vi "Lvi Read U32Data2D.vi"(0 "DataBufSize":u32, 1 "timeout":dbl, 5 "TaskRef":i32, 7 "PointsPerChan":u32, 9 "NumChansToRead":u32, 11 "error in (no error)":errorcluster, 12 "OnlyReadAvailable":bool) -> (3 "DataBuf":u32[](array[numeric]), 4 "DataBufSize out":u32, 6 "TaskRef out":i32, 8 "PointsPerChan out":u32, 10 "NumChansToRead out":u32, 14 "function return":i32, 15 "error out":errorcluster)   [LabVIEW 2022 SP3, in "DtLvLink.lvlib"]
doc: "Calls directly into the entry points of the DLL of the Data Acq SDK to return a two-dimensional array of unsigned, 32-bit integers representing the data points from the specified task."
uses:
  DtLvLink.lvlib
  <userlib>/LV-Link3/DtLvLink_64.dll
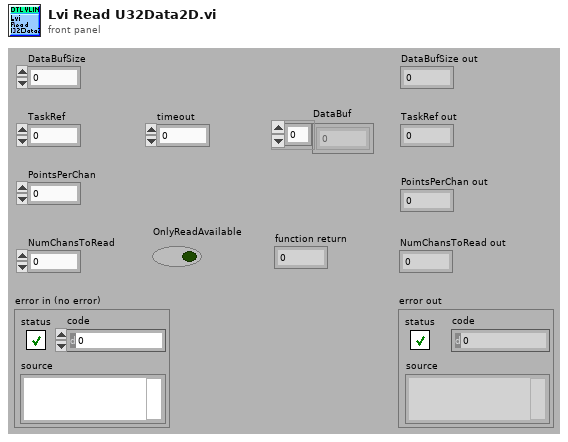
[diagram p1: front panel]
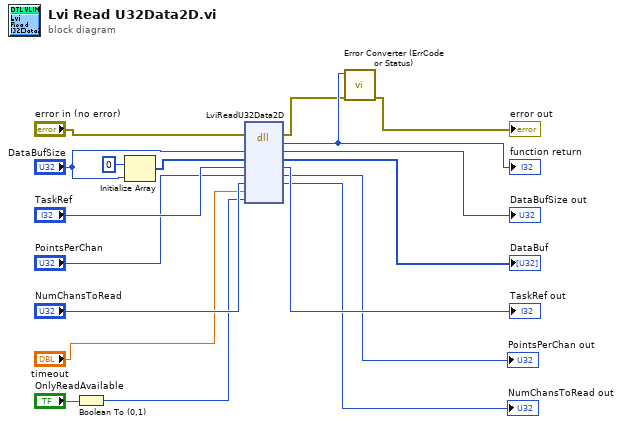
[diagram p0: block diagram]
diagram:
  n1 = Boolean To (0,1)(Boolean="OnlyReadAvailable") -> (0, 1=w3:i16)
  n2 = Initialize Array(u32 0 ("element"), "DataBufSize") -> (w15:u32[])
  n3 = dll-call lib="C:/Program Files/National Instruments/LabVIEW 2022/user.lib/LV-Link3/DtLvLink_64.*" fn="LviReadU32Data2D"(error in="error in (no error)", "DataBufSize"="DataBufSize", "DataBuf"=w15, "TaskRef"="TaskRef", "PointsPerChan"="PointsPerChan", "NumChansToRead"="NumChansToRead", "timeout"="timeout", "OnlyReadAvailable"=w3) -> (error out=w6:errorcluster, "return type"=w18:i32, "DataBufSize"=→"DataBufSize out":u32, "DataBuf"=→"DataBuf":u32[], "TaskRef"=→"TaskRef out":i32, "PointsPerChan"=→"PointsPerChan out":u32, "NumChansToRead"=→"NumChansToRead out":u32)  [unwired: 4 in, 1 out]
  "function return" <- w18
  n4 = call "Error Converter (ErrCode or Status).vi"("error in (no error)"=w6, "error code"=w18) -> ("error out"=→"error out":errorcluster)  [unwired: 9 in]
